vi "updateHelperText.vi"(8 "error in (no error)":errorcluster, 10 "Helper Text":string, 11 "Filled Text Fields Actor in":refnum<class "Filled Text Fields Actor.lvclass">) -> (0 "error out":errorcluster, 3 "Filled Text Fields Actor out":refnum<class "Filled Text Fields Actor.lvclass">)   [LabVIEW 2017, in "Filled Text Fields.lvlib" / "Filled Text Fields Actor.lvclass"]
uses:
  Filled Text Fields Actor.lvclass
  Filled Text Fields Actor.lvclass/Filled Text Fields Actor.ctl
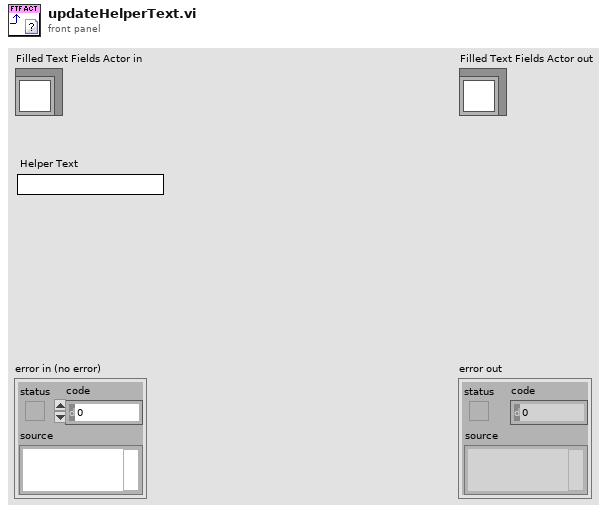
[diagram p1: front panel]
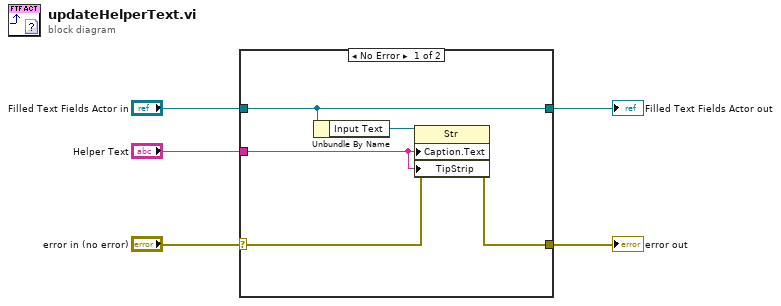
[diagram p0: block diagram]
diagram:
  n1 = case shown="No Error" "error in (no error)" {
    selector: "error in (no error)" -> [w8 w12]
    tunnel: [w7 w12] -> w4
    tunnel: [w10 w11] -> w2
    tunnel: "Filled Text Fields Actor in" -> [w10 w11]
    tunnel: "Helper Text" -> [w6 _]
    frame No Error {
      n2 = Unbundle By Name(w10) -> ("Input Text"=w9:refnum<vi>)
      n3 = property class="Str"(reference=w9, error in=w8, "Caption.Text"=w6, "TipStrip"=w6) -> (error out=w7:errorcluster)  [unwired: 1 out]
    }
    frame Error {
    }
  }
  "error out" <- w4
  "Filled Text Fields Actor out" <- w2
